vi "MAIN TRIAL CODE.vi"() -> ()   [LabVIEW 2025]
doc: "Use this template to build a producer/consumer design pattern with events to produce queue items. Use this design pattern instead of the User Interface Event Handler pattern for user interfaces when you want to execute code asynchronously in response to an event without slowing the user interface responsiveness."
panel:
  out "AE Ring-Down Counts":u32
  out "System Status":u32
  out "Timestamp":u32
  out "Sequence ID":u32
  out "Signal Energy":u32(graph)
  out "Amplitude db_AE":u32(graph)
  out "Peak Amplitude":u32(graph)
  in  "Uplink Packet":T1
  in  "Send Command":bool
  out "Isolated Gain":u32
  out "DAQ Status":u32
  in  "Connect Sensor":bool
  in  "stop":bool
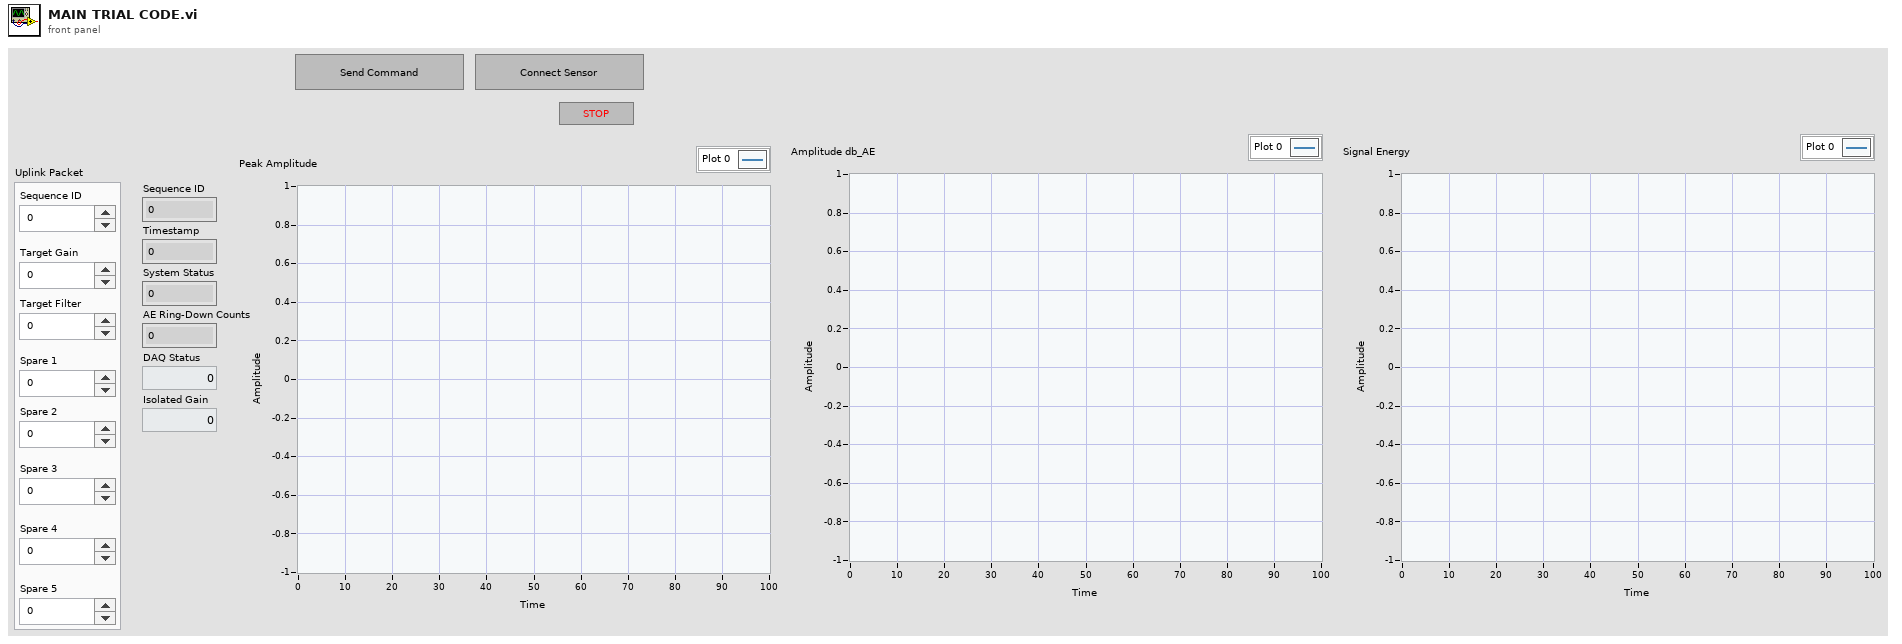
[diagram p1: front panel]
types:
  T1 = cluster{"Sequence ID":u32, "Target Gain":u32, "Target Filter":u32, "Spare 1":u32, "Spare 2":u32, "Spare 3":u32, "Spare 4":u32, "Spare 5":u32}
  T2 = cluster{"Sequence ID":u32, "Timestamp":u32, "System Status":u32, "Peak Amplitude":u32, "Amplitude dB_AE":u32, "AE Ring-Down Counts":u32, "Signal Energy":u32, "Spare 1":u32}
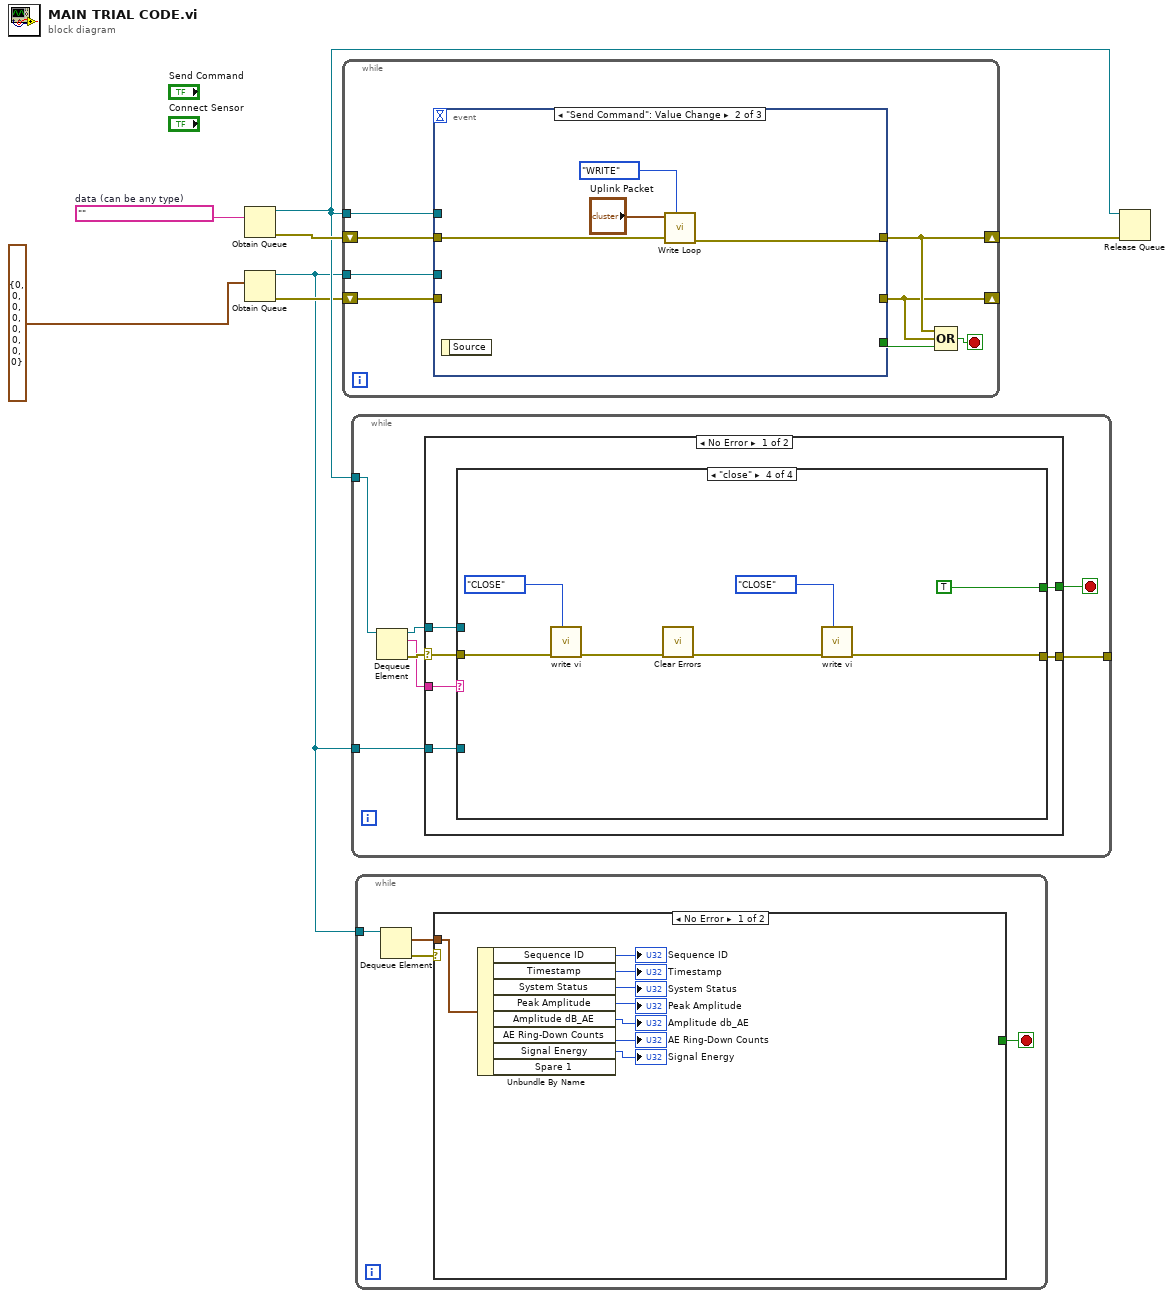
[diagram p0: block diagram]
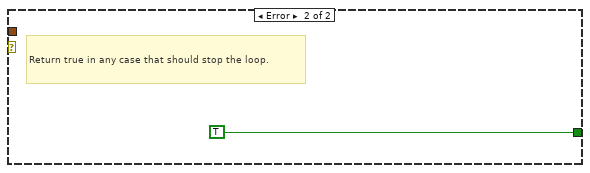
[diagram p2: hidden frame]
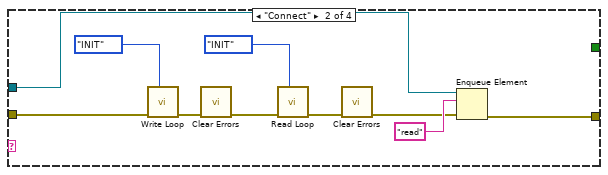
[diagram p4: hidden frame]
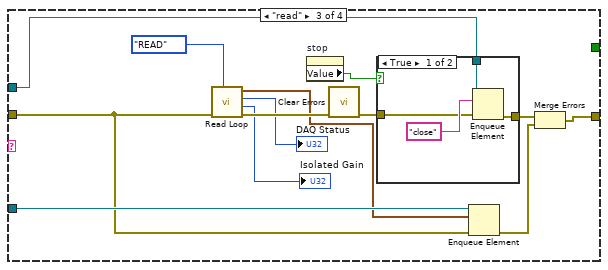
[diagram p5: hidden frame]
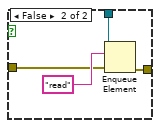
[diagram p6: hidden frame]
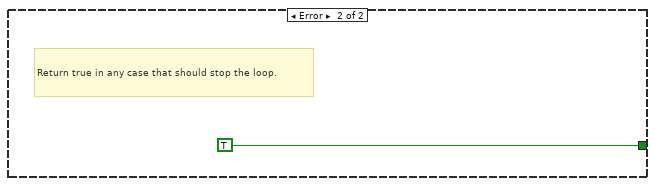
[diagram p7: hidden frame]
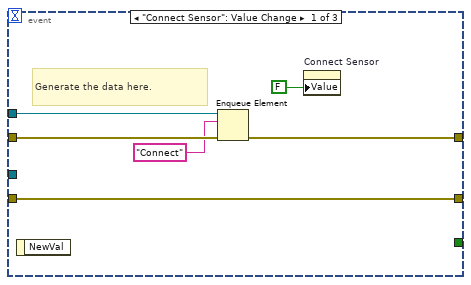
[diagram p8: hidden frame]
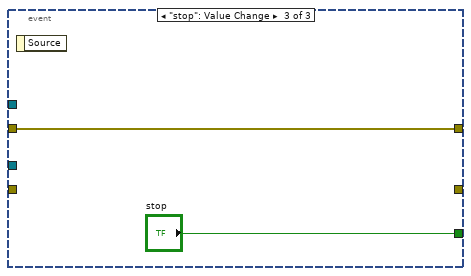
[diagram p9: hidden frame]
diagram:
  w5 = ""  # data (can be any type)
  n1 = Obtain Queue(element data type=w5) -> (queue out=w4:refnum<queue>, error out=w7:errorcluster)  [unwired: 4 in, 1 out]
  n2 = Obtain Queue(element data type=T2 {"Sequence ID"=0, "Timestamp"=0, "System Status"=0, "Peak Amplitude"=0, "Amplitude dB_AE"=0, "AE Ring-Down Counts"=0, "Signal Energy"=0, "Spare 1"=0} ("Downlink Packet")) -> (queue out=w2:refnum<queue>, error out=w3:errorcluster)  [unwired: 4 in, 1 out]
  n3 = while {
    shift-right: [w9] -> w6
    shift-left: w7 -> [w14]
    tunnel: w4 -> [w15]
    tunnel: w2 -> [w11]
    shift-right: [w8] -> _
    shift-left: w3 -> [w10]
    stop <- w12 stop-if-true
    n4 = event shown="[1] \"Send Command\": Value Change" {
      selector: _ -> [_ _ _]
      dyn-events: _ -> [_ _ _]
      timeout: _ -> [_ _ _]
      tunnel: w15 -> [w21 _ _]
      tunnel: w14 -> [w20 w25 w26]
      tunnel: [w19 w23 w26] -> w9
      tunnel: [_ _ "stop"] -> w13
      tunnel: w11 -> [_ _ _]
      tunnel: w10 -> [w17 _ _]
      tunnel: [w17 _ _] -> w8
      event "Connect Sensor": Value Change {
        # "Generate the data here."
        n5 = event-data() -> ()  [unwired: 1 in, 1 out]
        n6 = Enqueue Element(queue=w21, element="Connect", error in (no error)=w20) -> (error out=w19:errorcluster)  [unwired: 1 in, 2 out]
        n7 = property on="Connect Sensor" class="Bool (strict)"("Value"=FALSE ("Connect Sensor")) -> ()  [unwired: 2 in, 2 out]
      }
      event "Send Command": Value Change {
        n8 = event-data() -> ()  [unwired: 1 in, 1 out]
        n9 = call "Write Loop.vi"("Enum - Menu"=enum16{"INIT", "WRITE", "RE-INIT", "CLOSE"}."WRITE", "error in (no error)"=w25, "Uplink Packet"="Uplink Packet") -> ("error out"=w23:errorcluster)  [unwired: 8 in]
      }
      event "stop": Value Change {
        n10 = event-data() -> ()  [unwired: 1 in, 1 out]
      }
    }
    n11 = Compound Arithmetic op=OR(w9, w8, w13) -> (w12:bool)
  }
  n12 = while {
    tunnel: w4 -> [w34]
    tunnel: [w29] -> _
    tunnel: w2 -> [w28]
    stop <- w31 stop-if-true
    n13 = Dequeue Element(queue=w34) -> (queue out=w30:refnum<queue>, element=w32:string, error out=w33:errorcluster)  [unwired: 2 in, 1 out]
    n14 = case shown="No Error" w33 {
      selector: w33 -> [w38 _]
      tunnel: w32 -> [w40 _]
      tunnel: [w36 TRUE] -> w31
      tunnel: w30 -> [w39 _]
      tunnel: [w37 _] -> w29
      tunnel: w28 -> [w35 _]
      frame No Error {
        n15 = case shown="\"close\"" w40 {
          tunnel: w39 -> [_ w50 w63 _]
          tunnel: w38 -> [w41 w49 w55 w79]
          tunnel: [w41 w46 w54 w75] -> w37
          tunnel: [_ _ _ TRUE] -> w36
          tunnel: w35 -> [_ _ w57 _]
          frame "False", Default {
          }
          frame "Connect" {
            n16 = call "Write Loop.vi"("Enum - Menu"=enum16{"INIT", "WRITE", "RE-INIT", "CLOSE"}."INIT", "error in (no error)"=w49) -> ("error out"=w48:errorcluster)  [unwired: 9 in]
            n17 = call <vilib>:"Clear Errors.vi"("error in (no error)"=w48) -> ("error out"=w45:errorcluster)  [unwired: 5 in, 1 out]
            n18 = call "Read Loop.vi"("Enum - Menu"=enum16{"INIT", "READ", "RE-INIT", "CLOSE"}."INIT", "error in (no error)"=w45) -> ("error out"=w44:errorcluster)  [unwired: 6 in, 3 out]
            n19 = call <vilib>:"Clear Errors.vi"("error in (no error)"=w44) -> ("error out"=w42:errorcluster)  [unwired: 5 in, 1 out]
            n20 = Enqueue Element(queue=w50, element="read", error in (no error)=w42) -> (error out=w46:errorcluster)  [unwired: 1 in, 2 out]
          }
          frame "read" {
            n21 = call "Read Loop.vi"("Enum - Menu"=enum16{"INIT", "READ", "RE-INIT", "CLOSE"}."READ", "error in (no error)"=w55) -> ("error out"=w62:errorcluster, "Isolated Gain"=→"Isolated Gain":u32, "DAQ Status"=→"DAQ Status":u32, "Downlink Packet"=w56:T2)  [unwired: 6 in]
            n22 = property on="stop" class="Bool (strict)"() -> ("Value"=w60:bool)  [unwired: 2 in, 2 out]
            n23 = call <vilib>:"Clear Errors.vi"("error in (no error)"=w62) -> ("error out"=w52:errorcluster)  [unwired: 5 in, 1 out]
            n24 = case shown="True" w60 {
              tunnel: [w67 w71] -> w64
              tunnel: w63 -> [w66 w70]
              tunnel: w52 -> [w65 w69]
              frame True {
                n25 = Enqueue Element(queue=w66, element="close", error in (no error)=w65) -> (error out=w67:errorcluster)  [unwired: 1 in, 2 out]
              }
              frame False {
                n26 = Enqueue Element(queue=w70, element="read", error in (no error)=w69) -> (error out=w71:errorcluster)  [unwired: 1 in, 2 out]
              }
            }
            n27 = Enqueue Element(queue=w57, element=w56, error in (no error)=w55) -> (error out=w53:errorcluster)  [unwired: 1 in, 2 out]
            n28 = Merge Errors(w64, w53) -> (w54:errorcluster)
          }
          frame "close" {
            n29 = call "write vi.vi"("Enum - Menu"=enum16{"INIIT", "WRITE", "REINT", "CLOSE"}."CLOSE", "error in (no error)"=w79) -> ("error out"=w77:errorcluster)  [unwired: 8 in, 1 out]
            n30 = call <vilib>:"Clear Errors.vi"("error in (no error)"=w77) -> ("error out"=w73:errorcluster)  [unwired: 5 in, 1 out]
            n31 = call "write vi.vi"("Enum - Menu"=enum16{"INIIT", "WRITE", "REINT", "CLOSE"}."CLOSE", "error in (no error)"=w73) -> ("error out"=w75:errorcluster)  [unwired: 8 in, 1 out]
          }
        }
      }
      frame Error {
        # "Return true in any case that should stop the loop."
      }
    }
  }
  n32 = while {
    tunnel: w2 -> [w84]
    stop <- w81 stop-if-true
    n33 = Dequeue Element(queue=w84) -> (element=w82:T2, error out=w83:errorcluster)  [unwired: 2 in, 2 out]
    n34 = case shown="No Error" w83 {
      tunnel: w82 -> [w92 _]
      tunnel: [_ TRUE] -> w81
      frame No Error {
        n35 = Unbundle By Name(w92) -> ("Sequence ID"=→"Sequence ID":u32, "Timestamp"=→"Timestamp":u32, "System Status"=→"System Status":u32, "Peak Amplitude"=→"Peak Amplitude":u32, "Amplitude dB_AE"=→"Amplitude db_AE":u32, "AE Ring-Down Counts"=→"AE Ring-Down Counts":u32, "Signal Energy"=→"Signal Energy":u32)  [unwired: 1 out]
      }
      frame Error {
        # "Return true in any case that should stop the loop."
      }
    }
  }
  n36 = Release Queue(queue=w4, error in (no error)=w6) -> ()  [unwired: 1 in, 3 out]
